vi "nanocal -- tensors and stuff -- V1.vi"(6 "parameters IN":map{T1, dbl}(c390), 7 "action":T2=enum."onlygrads", 8 "d2G / d log λ1 d log λ2  = ⟨ λ1 dζ(ω)/dλ1 | λ2 dζ(ω)/dλ2 ⟩":map{T1[], dbl}(c390), 9 "G":dbl=-1.0, 10 "dG / dlog λ  =  ⟨ (ξ(ω)-ζ(ω)) | λdζ(ω)/dλ ⟩":map{T1, dbl}(c390), 11 "parameter tensor order IN":map{i32, T1}(c390)) -> (0 "vector dlogG / d log a   out":dbl[](array[numeric]), 1 "map1 out":map{T1, dbl}(c390), 2 "map2 out":map{T1, dbl}(c390))   [LabVIEW 2021]
uses:
  3-lorentzian-parameters.ctl
  3-lorentzian-heat-response action.ctl
  <vilib>/Utility/miscctls.llb/LVMapReplaceAction.ctl
  <vilib>/Analysis/baseanly.llb/Matrix Type of Inverse Matrix.ctl
  <vilib>/Analysis/baseanly.llb/Real A x B.vi
  <vilib>/Analysis/Matrix/Numeric/Conversions/Array To Matrix - RA2.vi
  <vilib>/Analysis/baseanly.llb/Real Inverse Matrix.vi
  <vilib>/Analysis/Matrix/Numeric/Conversions/Matrix To Array - RM.vi
  <vilib>/Analysis/Matrix/Numeric/Conversions/Array To Matrix - RA.vi
  <vilib>/Analysis/7linalg.llb/Solve Linear Equations (multiple right hand).vi
  <vilib>/Analysis/Matrix/NI_Matrix.lvlib
  <vilib>/Analysis/NI_AALBase.lvlib
  <vilib>/Analysis/NI_AALPro.lvlib
panel:
  out "ζ(ω) out":cdb[](array[numeric])=[1.7183506006211996e-05+0.0i, 1.7124360968751133e-05+0.0i, 1.7049104347380084e-05+0.0i, 1.700437896335042e-05+0.0i, 1.6984579723285106e-05+0.0i, 1.702277369054923e-05+0.0i, 1.713094025845651e-05+0.0i, 1.734249707866828e-05+0.0i, 1.768320429215342e-05+0.0i, 1.8195281152538477e-05+0.0i, 1.8917228661806973e-05+0.0i, 1.9897834564883332e-05+0.0i, 2.154104046962704e-05+0.0i, 2.3247799321765792e-05+0.0i, 2.5364678450551808e-05+0.0i, 2.8645788781885885e-05+0.0i, 3.204749554800641e-05+0.0i, 3.783559691555022e-05+0.0i, 4.245015867332296e-05+0.0i, 4.909131821431355e-05+0.0i, 5.511821898441184e-05+0.0i, 6.178843506022867e-05+0.0i, 7.1079604965352e-05+0.0i, 7.922304381453334e-05+0.0i, 8.814778883893872e-05+0.0i, 9.806709148886077e-05+0.0i, 0.00011119043245647465+0.0i, 0.00012253184919712196+0.0i, 0.00013777724317049346+0.0i, 0.0001508081004573332+0.0i, 0.00016547294918783876+0.0i, 0.00018003847596605868+0.0i, 0.00019518361086534857+0.0i, 0.00021134179818259658+0.0i, 0.0002372041782935464+0.0i, 0.00025518143132024254+0.0i, 0.0002835129702467886+0.0i, 0.0003060118087631287+0.0i, 0.00032860772064336976+0.0i, 0.0003492674091322389+0.0i, 0.00037498324855458583+0.0i, 0.00040021078021115026+0.0i, 0.00041969942568205823+0.0i, 0.00044367338947118773+0.0i, 0.0004634793607238068+0.0i, 0.00047921028781215815+0.0i, 0.0004880906353641744+0.0i, 0.0004932212623741357+0.0i, 0.000491476456593048+0.0i, 0.000480893803992059+0.0i, 0.0004535995818650303+0.0i, 0.000417087772881063+0.0i, 0.0003564148692854789+0.0i, 0.0003049201646356487+0.0i, 0.00021260191240459413+0.0i, 0.00011714858948470126+0.0i, 1.675457544365132e-05+0.0i, -6.8674075405897e-05+0.0i, -0.000156473047607305+0.0i, -0.00026709373934749337+0.0i, -0.0003544271565676041+0.0i, -0.00047937600197311275+0.0i, -0.0006086290582260493+0.0i, -0.0007031877411848573+0.0i, -0.0007564526901441745+0.0i, -0.000802489180995596+0.0i, -0.0008414596018105983+0.0i, -0.0008809346482248761+0.0i, -0.0009073902840241921+0.0i, -0.0009264953054508651+0.0i, -0.0009405659412141811+0.0i, -0.000951649722530156+0.0i, -0.0009557485581057351+0.0i, -0.0009558464741053665+0.0i, -0.0009509110176922098+0.0i, -0.0009411315169847015+0.0i, -0.0009303400913929496+0.0i, -0.0009171113529290538+0.0i, -0.0009022111527275027+0.0i, -0.0008813746494947608+0.0i, -0.0008581837971946129+0.0i, -0.0008372063466683705+0.0i, -0.0008165626610594428+0.0i, -0.0007901155435838691+0.0i, -0.0007682834352800848+0.0i, -0.000746231015527196+0.0i, -0.0007238798463130141+0.0i, -0.0007015567569177018+0.0i, -0.000679301954671598+0.0i, -0.0006572001413831251+0.0i, -0.000629855254567978+0.0i, -0.0006083942229188815+0.0i, -0.0005768631156754208+0.0i, -0.0005562177438951648+0.0i, -0.0005359092039599222+0.0i, -0.0005145186443378148+0.0i, -0.0004951602053444319+0.0i, -0.00047624970229075174+0.0i, -0.0004577401041527736+0.0i, -0.00043519037796120065+0.0i]
  out "ζ(ω) norm":dbl=-1.0
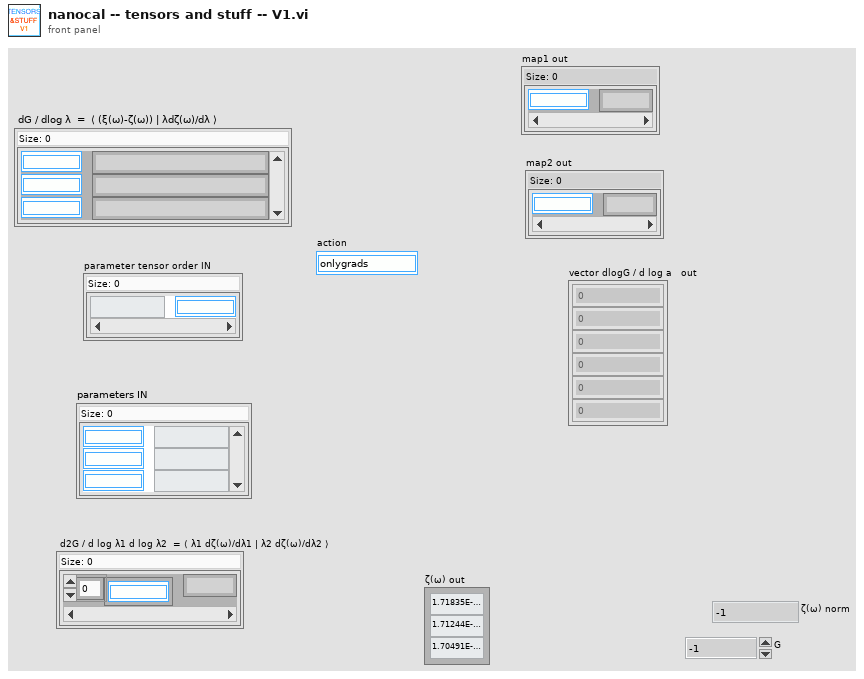
[diagram p1: front panel]
types:
  T1 = typedef "3-lorentzian-parameters.ctl" = enum16{"ζ", "τ1", "τS", "τN", "τC", "κ0", "m1", "m2", "m3", "T (K)", "B (T)", "θ (deg)", "side (S|R)", "set of (B|T)", "Re(offset)", "Im(offset)", "στ1", "στ1-", "στ1+", "στS", "στS-", "στS+", "στN", "στN-", "στN+", "τ11", "τ12", "τ21", "τ22", "τN1", "τN2"}
  T2 = typedef "3-lorentzian-heat-response action.ctl" = enum16{"calc R", "create string", "calc m1m2m3", "dζ", "dT1", "dτS", "dτN", "dτC", "d-all", "dκ0", "T(K)", "m1", "m2", "m3", "parse string", "θ (deg)", "B (T)", "onlygrads", "newton", "create emty string", "simple2nd", "calc R2", "ScalarProd", "ScalarProd-diff", "nothing", "ScalarProd-eta", "tolog", "ignore", "three2nd", "eta-errors"}
  T3 = typedef "LVMapReplaceAction.ctl" = enum32{"Modify Entry only if found", "Add or Modify Entry", "Delete Entry"}
  T4 = typedef "NI_AALBase.lvlib/Matrix Type of Inverse Matrix.ctl" = enum32{"General", "Positive Definite", "Lower Triangular", "Upper Triangular"}
  T5 = typedef "NI_Matrix.lvlib/RealMatrix.ctl" = dbl[][]
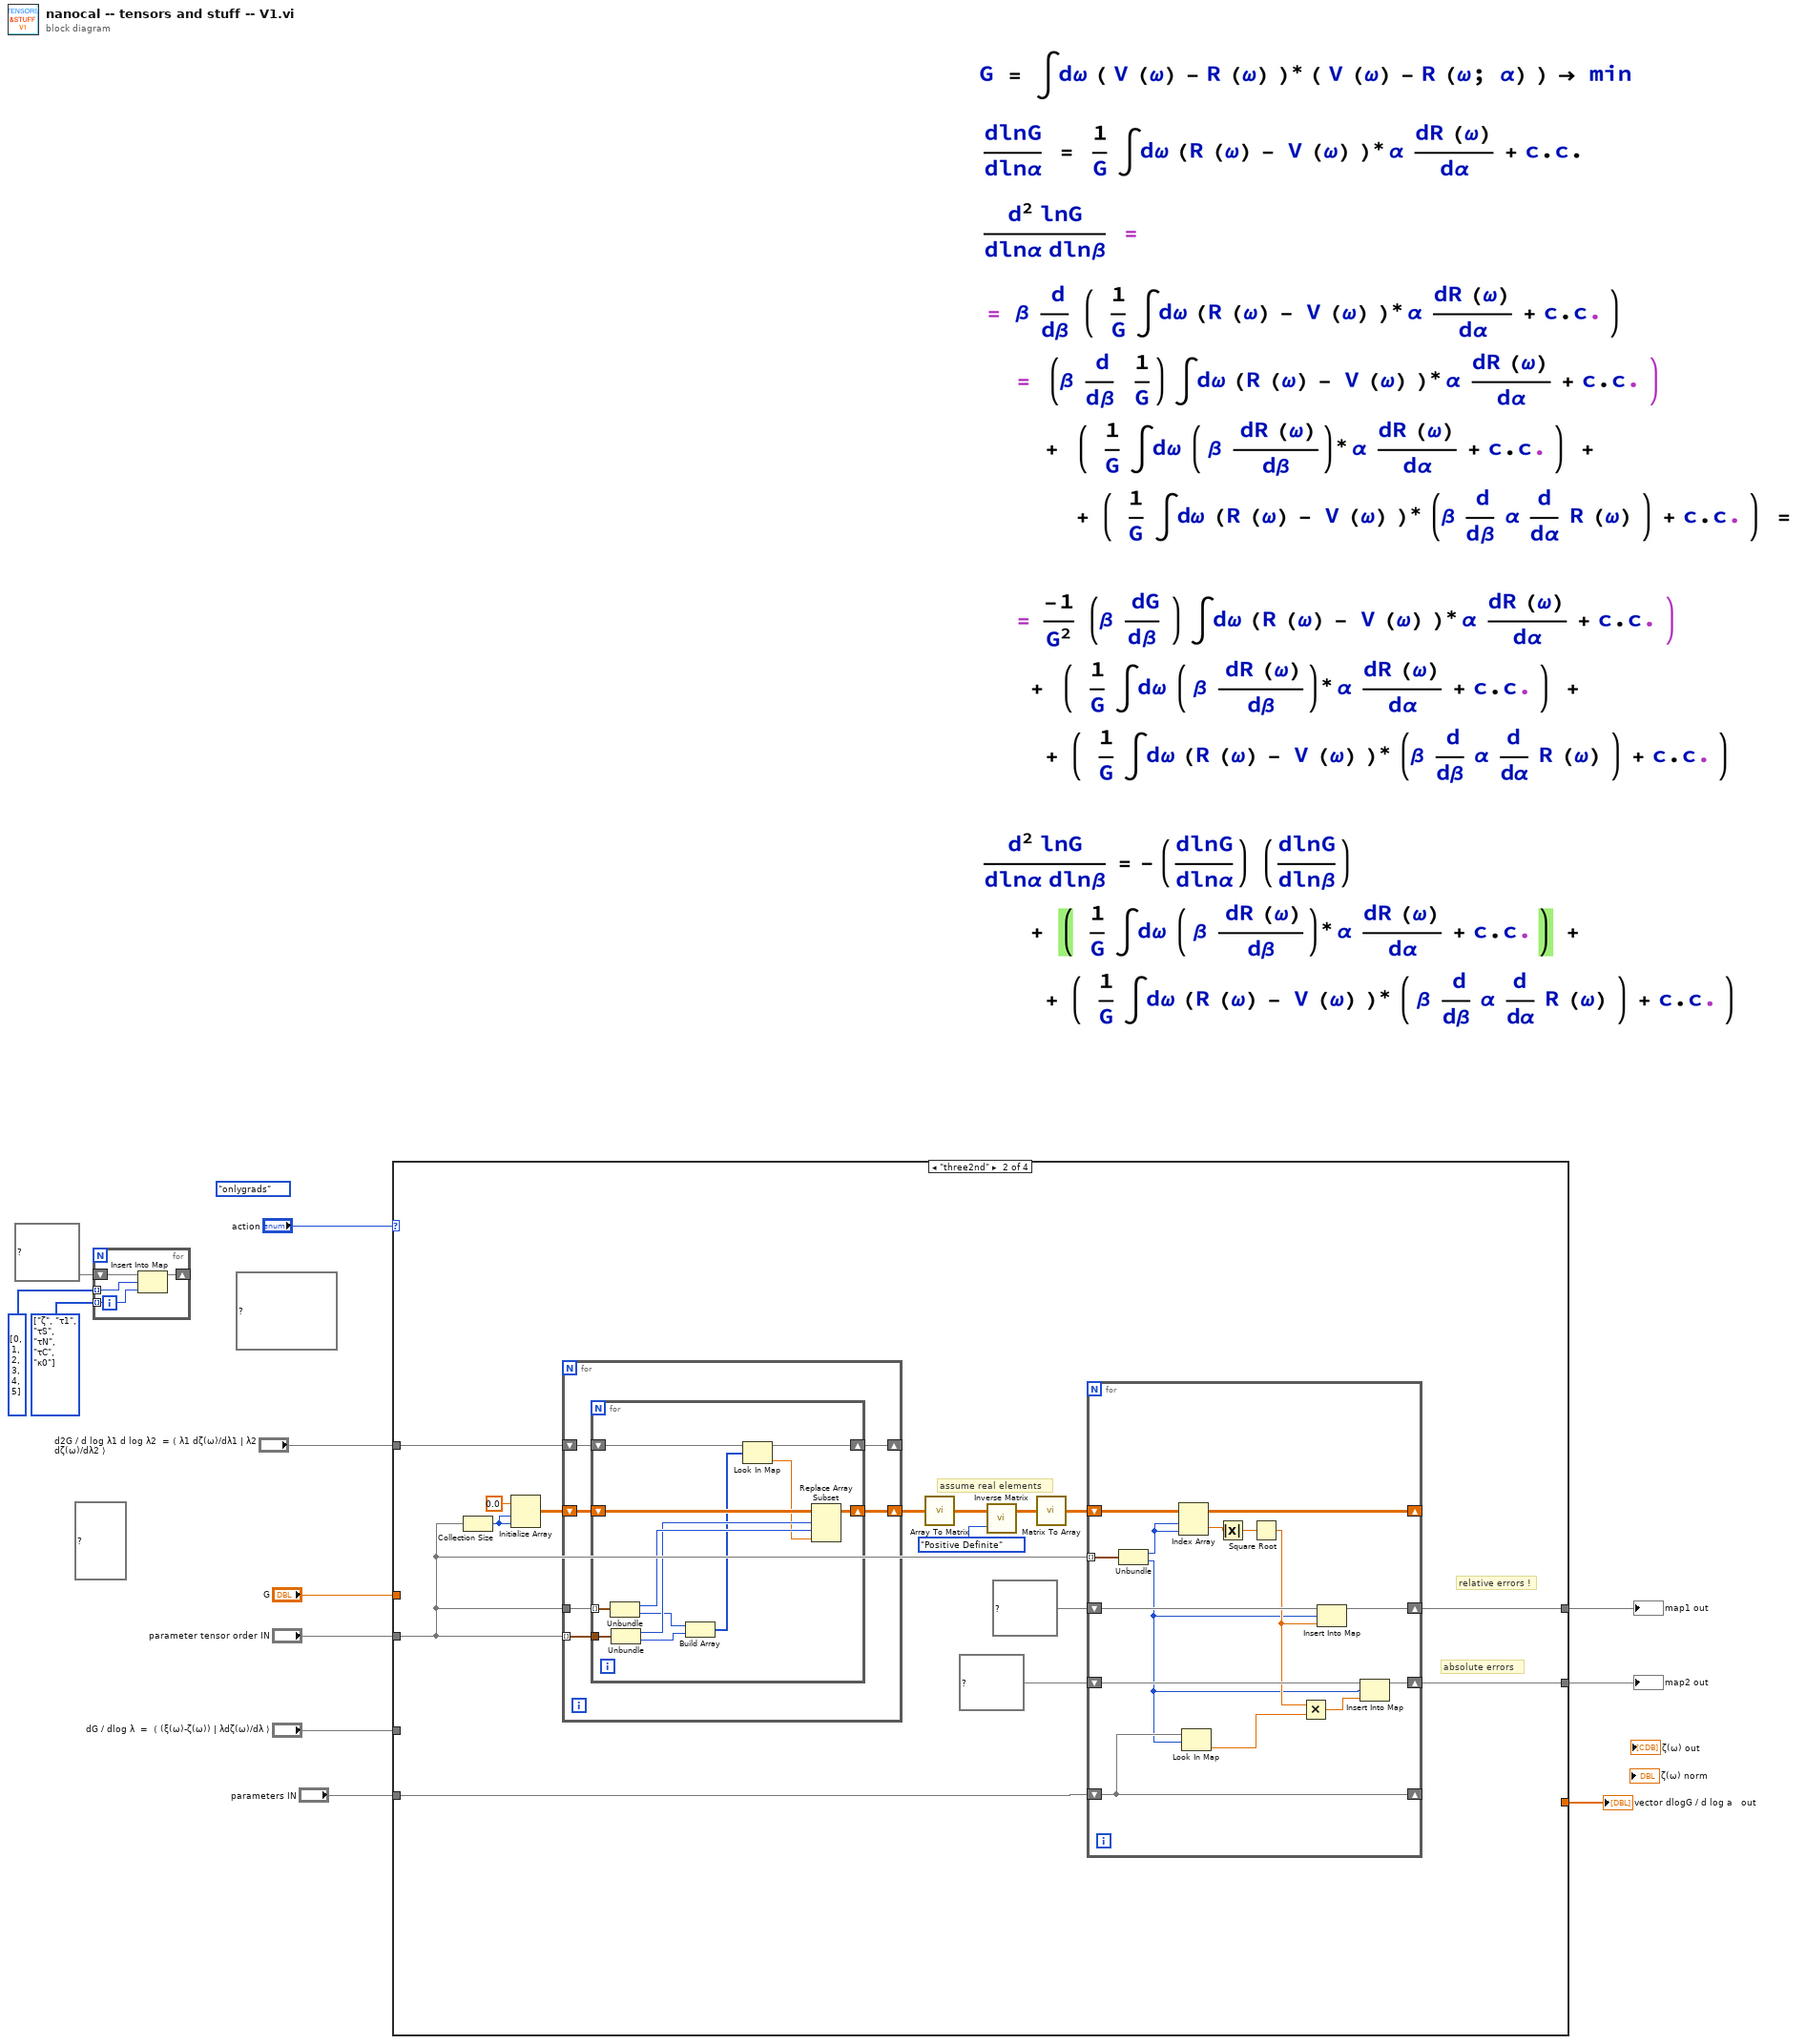
[diagram p0: block diagram]
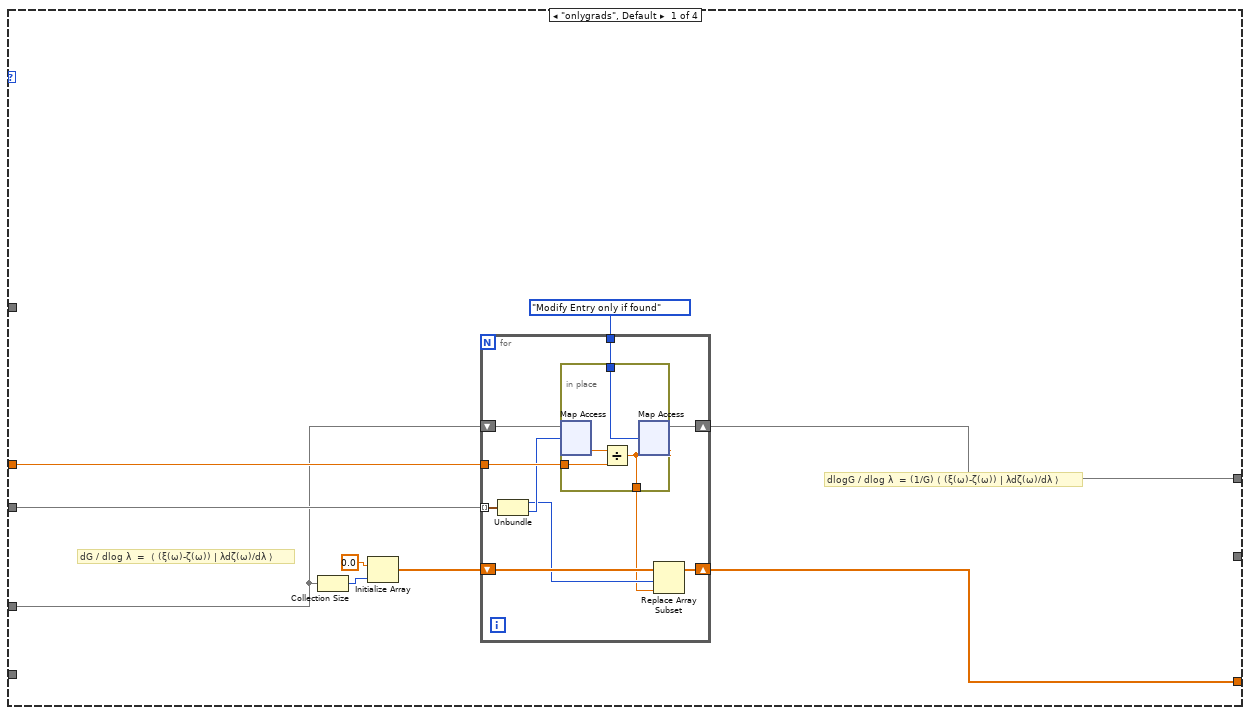
[diagram p2: hidden frame]
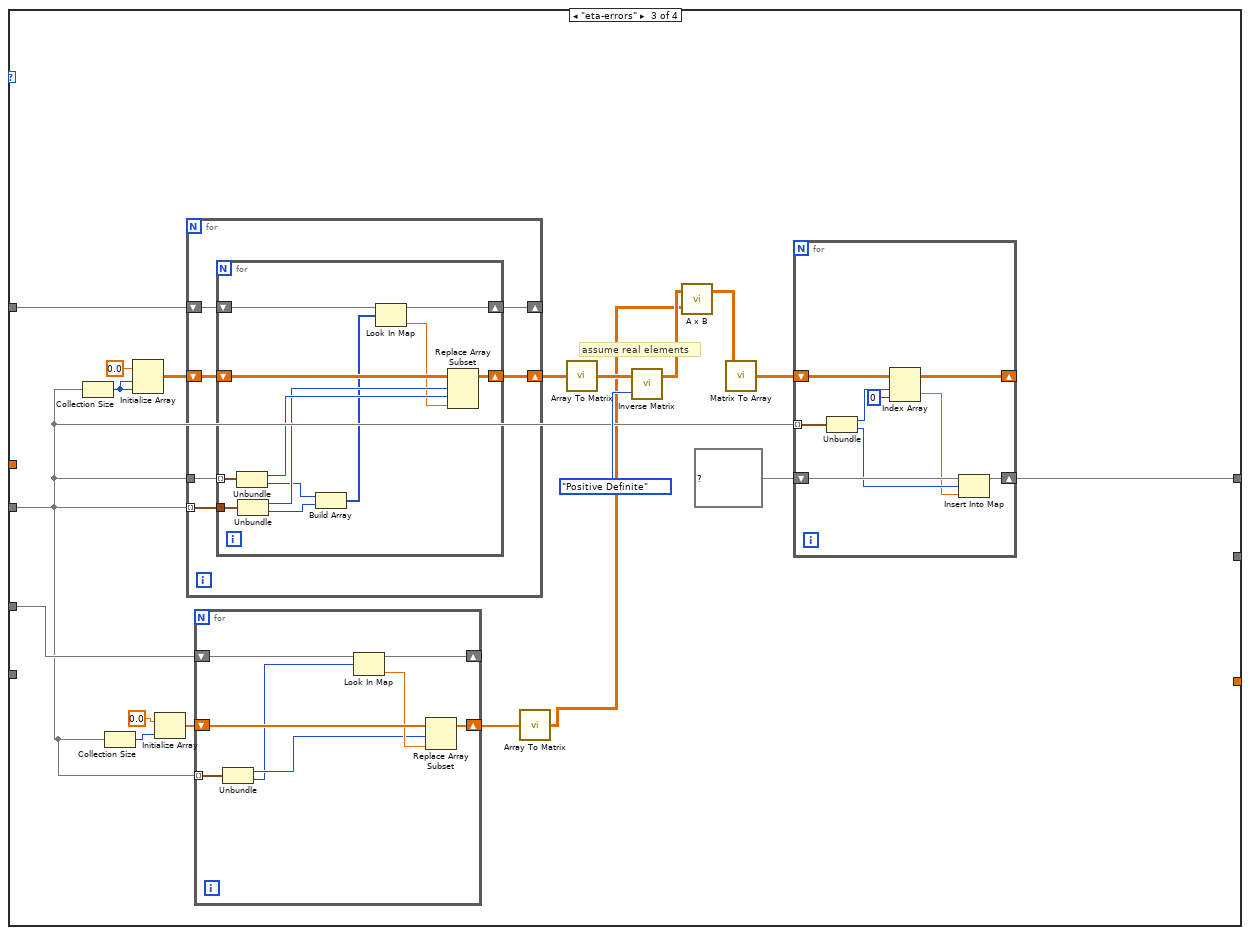
[diagram p3: hidden frame]
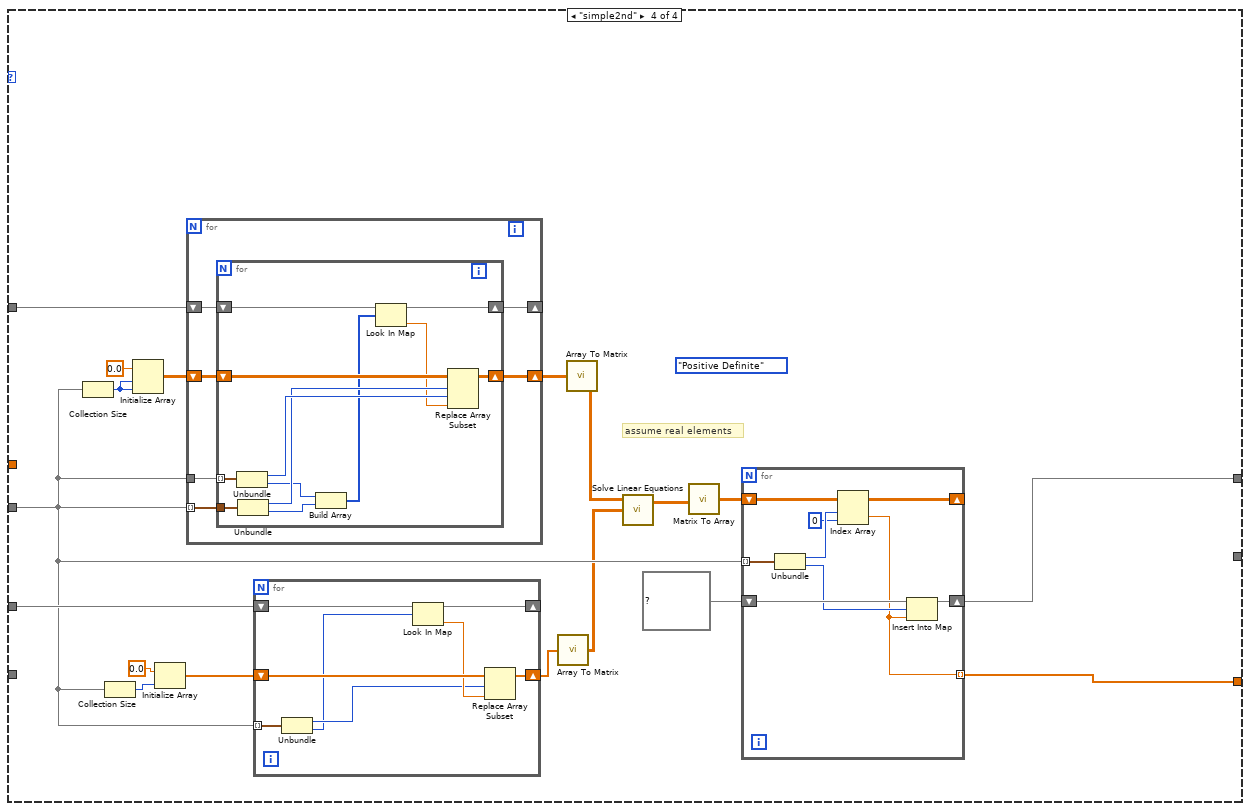
[diagram p4: hidden frame]
diagram:
  (unwired) map{T1[], dbl} {} ("d2G / d log λ1 d log λ2  = ⟨ λ1 dζ(ω)/dλ1 | λ2 dζ(ω)/dλ2 ⟩")
  (unwired) map{i32[], dbl} {} ("parameters IN")
  w7 = T1[] [enum."ζ", enum."τ1", enum."τS", enum."τN", enum."τC", enum."κ0"] items=["ζ", "τ1", "τS", "τN", "τC", "κ0", "m1", "m2", "m3", "T (K)", "B (T)", "θ (deg)", "side (S|R)", "set of (B|T)", "Re(offset)", "Im(offset)", "στ1", "στ1-", "στ1+", "στS", "στS-", "στS+", "στN", "στN-", "στN+", "τ11", "τ12", "τ21", "τ22", "τN1", "τN2"]
  (unwired) 3-lorentzian-heat-response_action."onlygrads" ("action")
  n1 = for {
    tunnel: w7 -> [w13] mode=indexing
    shift-right: [w15] -> _
    shift-left: map{i32, T1} {} ("parameters IN") -> [w16]
    tunnel: i32[] [0, 1, 2, 3, 4, 5] -> [w14] mode=indexing
    n2 = Insert Into Map(map in=w16, key=w14, value=w13) -> (map out=w15:map{i32, T1})  [unwired: 2 out]
  }
  n3 = case shown="\"three2nd\"" "action" {
    tunnel: "d2G / d log λ1 d log λ2  = ⟨ λ1 dζ(ω)/dλ1 | λ2 dζ(ω)/dλ2 ⟩" -> [_ w51 w101 w151]
    tunnel: "parameter tensor order IN" -> [w25 w46 w90 w142]
    tunnel: "dG / dlog λ  =  ⟨ (ξ(ω)-ζ(ω)) | λdζ(ω)/dλ ⟩" -> [w19 _ w94 w147]
    tunnel: "G" -> [w24 _ _ _]
    tunnel: [w22 w43 w95 w148] -> w4
    tunnel: [w17 _ _ w137] -> w3
    tunnel: "parameters IN" -> [_ w41 _ _]
    tunnel: [_ w40 _ _] -> w1
    frame "onlygrads", Default {
      # "dlogG / dlog λ  = (1/G) ⟨ (ξ(ω)-ζ(ω)) | λdζ(ω)/dλ ⟩"
      # "dG / dlog λ  =  ⟨ (ξ(ω)-ζ(ω)) | λdζ(ω)/dλ ⟩"
      n4 = Collection Size(1:w19) -> (0:w20:i32)
      n5 = Initialize Array(0.0 ("element"), w20) -> (w18:dbl[])
      n6 = for {
        tunnel: w25 -> [w32] mode=indexing
        shift-right: [w34] -> w22
        shift-left: w19 -> [w35]
        tunnel: w24 -> [w33]
        tunnel: LVMapReplaceAction."Modify Entry only if found" ("action") -> [w30]
        shift-right: [w28] -> w17
        shift-left: w18 -> [w29]
        n7 = Unbundle(w32) -> ("index"=w27:i32, "X selector"=w31:T1)
        n8 = in-place {
          in-place-border: w33 -> [w38]
          in-place-border: w30 -> [w37]
          in-place-border: [w36] -> w26
          n9 = in-place-map #1(w35, w31) -> (w39:dbl)  [unwired: 1 in, 1 out]
          n10 = Divide(x=w39, y=w38) -> (x/y=w36:dbl)
          n11 = in-place-map #1(w36, w37) -> (w34:map{T1, dbl})  [unwired: 2 out]
        }
        n12 = Replace Array Subset(array=w29, new element=w26, index=w27) -> (w28:dbl[])
      }
    }
    frame "three2nd" {
      # "absolute errors"
      # "relative errors !"
      # "assume real elements"
      n13 = Collection Size(1:w46) -> (0:w53:i32)
      n14 = Initialize Array(0.0 ("element"), w53, w53) -> (w52:dbl[][])
      n15 = for {
        tunnel: w46 -> [w74] mode=indexing
        tunnel: w46 -> [w73]
        shift-right: [w71] -> w50
        shift-left: w52 -> [w72]
        shift-right: [w69] -> _
        shift-left: w51 -> [w70]
        n16 = for {
          tunnel: w74 -> [w85]
          tunnel: w73 -> [w84] mode=indexing
          shift-right: [w82] -> w71
          shift-left: w72 -> [w83]
          shift-right: [w76] -> w69
          shift-left: w70 -> [w76]
          n17 = Unbundle(w84) -> ("index"=w81:i32, "X selector"=w79:T1)
          n18 = Unbundle(w85) -> ("index"=w80:i32, "X selector"=w78:T1)
          n19 = Build Array(w79, w78) -> (w77:T1[])
          n20 = Look In Map(map=w76, key=w77) -> (value=w75:dbl)  [unwired: 1 in, 1 out]
          n21 = Replace Array Subset(array=w83, new element=w75, index (row)=w80, index (col)=w81) -> (w82:dbl[][])
        }
      }
      n22 = call-poly <vilib>:"Array To Matrix.vi"("Real 2D Array"=w50) -> ("Real Matrix"=w49:T5)
      n23 = call-poly <vilib>:"Inverse Matrix.vi"("matrix type"=Matrix_Type_of_Inverse_Matrix."Positive Definite", "Input Matrix"=w49) -> ("Inverse Matrix"=w47:T5)  [unwired: 1 out]
      n24 = call-poly <vilib>:"Matrix To Array.vi"("Real Matrix"=w47) -> ("Real 2D Array"=w45:dbl[][])
      n25 = for {
        tunnel: w46 -> [w67] mode=indexing
        shift-right: [w68] -> _
        shift-left: w45 -> [w68]
        shift-right: [w64] -> w43
        shift-left: map{T1, dbl} {} ("parameters IN") -> [w65]
        shift-right: [w60] -> w40
        shift-left: map{T1, dbl} {} ("parameters IN") -> [w61]
        shift-right: [w59] -> _
        shift-left: w41 -> [w59]
        n26 = Unbundle(w67) -> ("index"=w66:i32, "X selector"=w56:T1)
        n27 = Index Array(array=w68, index (row)=w66, index (col)=w66) -> (element=w63:dbl)
        n28 = Look In Map(map=w59, key=w56) -> (value=w58:dbl)  [unwired: 1 in, 1 out]
        n29 = Absolute Value(x=w63) -> (abs(x)=w62:dbl)
        n30 = Square Root(x=w62) -> (sqrt(x)=w57:dbl)
        n31 = Multiply(x=w57, y=w58) -> (x*y=w55:dbl)
        n32 = Insert Into Map(map in=w65, key=w56, value=w57) -> (map out=w64:map{T1, dbl})  [unwired: 2 out]
        n33 = Insert Into Map(map in=w61, key=w56, value=w55) -> (map out=w60:map{T1, dbl})  [unwired: 2 out]
      }
    }
    frame "eta-errors" {
      # "assume real elements"
      n34 = Collection Size(1:w90) -> (0:w103:i32)
      n35 = Collection Size(1:w90) -> (0:w92:i32)
      n36 = Initialize Array(0.0 ("element"), w103, w103) -> (w102:dbl[][])
      n37 = Initialize Array(0.0 ("element"), w92) -> (w91:dbl[])
      n38 = for {
        tunnel: w90 -> [w125] mode=indexing
        tunnel: w90 -> [w124]
        shift-right: [w122] -> w100
        shift-left: w102 -> [w123]
        shift-right: [w120] -> _
        shift-left: w101 -> [w121]
        n39 = for {
          tunnel: w125 -> [w136]
          tunnel: w124 -> [w135] mode=indexing
          shift-right: [w133] -> w122
          shift-left: w123 -> [w134]
          shift-right: [w127] -> w120
          shift-left: w121 -> [w127]
          n40 = Unbundle(w135) -> ("index"=w132:i32, "X selector"=w130:T1)
          n41 = Unbundle(w136) -> ("index"=w131:i32, "X selector"=w129:T1)
          n42 = Build Array(w130, w129) -> (w128:T1[])
          n43 = Look In Map(map=w127, key=w128) -> (value=w126:dbl)  [unwired: 1 in, 1 out]
          n44 = Replace Array Subset(array=w134, new element=w126, index (row)=w131, index (col)=w132) -> (w133:dbl[][])
        }
      }
      n45 = for {
        shift-right: [w110] -> w89
        shift-left: w91 -> [w111]
        shift-right: [w109] -> _
        shift-left: w94 -> [w109]
        tunnel: w90 -> [w107] mode=indexing
        n46 = Unbundle(w107) -> ("index"=w106:i32, "X selector"=w105:T1)
        n47 = Look In Map(map=w109, key=w105) -> (value=w108:dbl)  [unwired: 1 in, 1 out]
        n48 = Replace Array Subset(array=w111, new element=w108, index=w106) -> (w110:dbl[])
      }
      n49 = call-poly <vilib>:"Array To Matrix.vi"("Real 1D Array"=w89) -> ("Real Matrix (Column Vector)"=w87:T5)
      n50 = call-poly <vilib>:"Array To Matrix.vi"("Real 2D Array"=w100) -> ("Real Matrix"=w99:T5)
      n51 = call-poly <vilib>:"Inverse Matrix.vi"("matrix type"=Matrix_Type_of_Inverse_Matrix."Positive Definite", "Input Matrix"=w99) -> ("Inverse Matrix"=w88:T5)  [unwired: 1 out]
      n52 = call-poly <vilib>:"A x B.vi"("B"=w87, "A"=w88) -> ("A x B"=w86:T5)  [unwired: 1 out]
      n53 = call-poly <vilib>:"Matrix To Array.vi"("Real Matrix"=w86) -> ("Real 2D Array"=w97:dbl[][])
      n54 = for {
        tunnel: w90 -> [w118] mode=indexing
        shift-right: [w119] -> _
        shift-left: w97 -> [w119]
        shift-right: [w115] -> w95
        shift-left: map{T1, dbl} {} ("parameters IN") -> [w116]
        n55 = Unbundle(w118) -> ("index"=w117:i32, "X selector"=w114:T1)
        n56 = Index Array(array=w119, index (row)=w117, index (col)=0 ("disabled index (col)")) -> (element=w112:dbl)
        n57 = Insert Into Map(map in=w116, key=w114, value=w112) -> (map out=w115:map{T1, dbl})  [unwired: 2 out]
      }
    }
    frame "simple2nd" {
      (unwired) Matrix_Type_of_Inverse_Matrix."Positive Definite" ("matrix type")
      # "assume real elements"
      n58 = Collection Size(1:w142) -> (0:w153:i32)
      n59 = Collection Size(1:w142) -> (0:w145:i32)
      n60 = Initialize Array(0.0 ("element"), w153, w153) -> (w152:dbl[][])
      n61 = Initialize Array(0.0 ("element"), w145) -> (w144:dbl[])
      n62 = for {
        tunnel: w142 -> [w175] mode=indexing
        tunnel: w142 -> [w174]
        shift-right: [w172] -> w141
        shift-left: w152 -> [w173]
        shift-right: [w170] -> _
        shift-left: w151 -> [w171]
        n63 = for {
          tunnel: w175 -> [w186]
          tunnel: w174 -> [w185] mode=indexing
          shift-right: [w183] -> w172
          shift-left: w173 -> [w184]
          shift-right: [w177] -> w170
          shift-left: w171 -> [w177]
          n64 = Unbundle(w185) -> ("index"=w182:i32, "X selector"=w180:T1)
          n65 = Unbundle(w186) -> ("index"=w181:i32, "X selector"=w179:T1)
          n66 = Build Array(w180, w179) -> (w178:T1[])
          n67 = Look In Map(map=w177, key=w178) -> (value=w176:dbl)  [unwired: 1 in, 1 out]
          n68 = Replace Array Subset(array=w184, new element=w176, index (row)=w181, index (col)=w182) -> (w183:dbl[][])
        }
      }
      n69 = for {
        shift-right: [w160] -> w143
        shift-left: w144 -> [w161]
        shift-right: [w159] -> _
        shift-left: w147 -> [w159]
        tunnel: w142 -> [w157] mode=indexing
        n70 = Unbundle(w157) -> ("index"=w156:i32, "X selector"=w155:T1)
        n71 = Look In Map(map=w159, key=w155) -> (value=w158:dbl)  [unwired: 1 in, 1 out]
        n72 = Replace Array Subset(array=w161, new element=w158, index=w156) -> (w160:dbl[])
      }
      n73 = call-poly <vilib>:"Array To Matrix.vi"("Real 1D Array"=w143) -> ("Real Matrix (Column Vector)"=w139:T5)
      n74 = call-poly <vilib>:"Array To Matrix.vi"("Real 2D Array"=w141) -> ("Real Matrix"=w140:T5)
      n75 = call-poly <vilib>:"Solve Linear Equations.vi"("Known Matrix"=w139, "Input Matrix"=w140) -> ("Solution Matrix"=w138:T5)  [unwired: 1 in, 1 out]
      n76 = call-poly <vilib>:"Matrix To Array.vi"("Real Matrix"=w138) -> ("Real 2D Array"=w150:dbl[][])
      n77 = for {
        tunnel: w142 -> [w168] mode=indexing
        shift-right: [w169] -> _
        shift-left: w150 -> [w169]
        shift-right: [w166] -> w148
        shift-left: map{T1, dbl} {} ("parameters IN") -> [w167]
        tunnel: [w162] -> w137 mode=indexing
        n78 = Unbundle(w168) -> ("index"=w164:i32, "X selector"=w165:T1)
        n79 = Index Array(array=w169, index (row)=w164, index (col)=0 ("disabled index (col)")) -> (element=w162:dbl)
        n80 = Insert Into Map(map in=w167, key=w165, value=w162) -> (map out=w166:map{T1, dbl})  [unwired: 2 out]
      }
    }
  }
  "map1 out" <- w4
  "vector dlogG / d log a   out" <- w3
  "map2 out" <- w1
